vi "stimulate_and_record.vi"(3 "SSH password":string, 4 "Transfer and Run Date Folder After Experiment":bool, 5 "SSH user name":string, 6 "Tags":string, 7 "Frames":i32, 8 "Convert Power to Voltage":bool, 9 "voltages/power":dbl[](array[numeric]), 10 "parameters":string[](array[string]), 11 "parameters headers":string[](array[string])) -> ()   [LabVIEW 2014]
uses:
  <vilib>/userdefined/High Color/IMAQdx.ctl
  <vilib>/Utility/file.llb/Write To Spreadsheet File (DBL).vi
  <vilib>/Utility/file.llb/Write To Spreadsheet File (string).vi
  <vilib>/Utility/file.llb/Read From Spreadsheet File (string).vi
  <vilib>/vision/driver/NI_Vision_Acquisition_Software.lvlib
panel:
  out "JPEG Quality":dbl
  out "Error":string
  out "Save Directory":path
  out "Buffer Number Out":u32
  out "Image":T1(plugin-control)
  in  "stop":bool
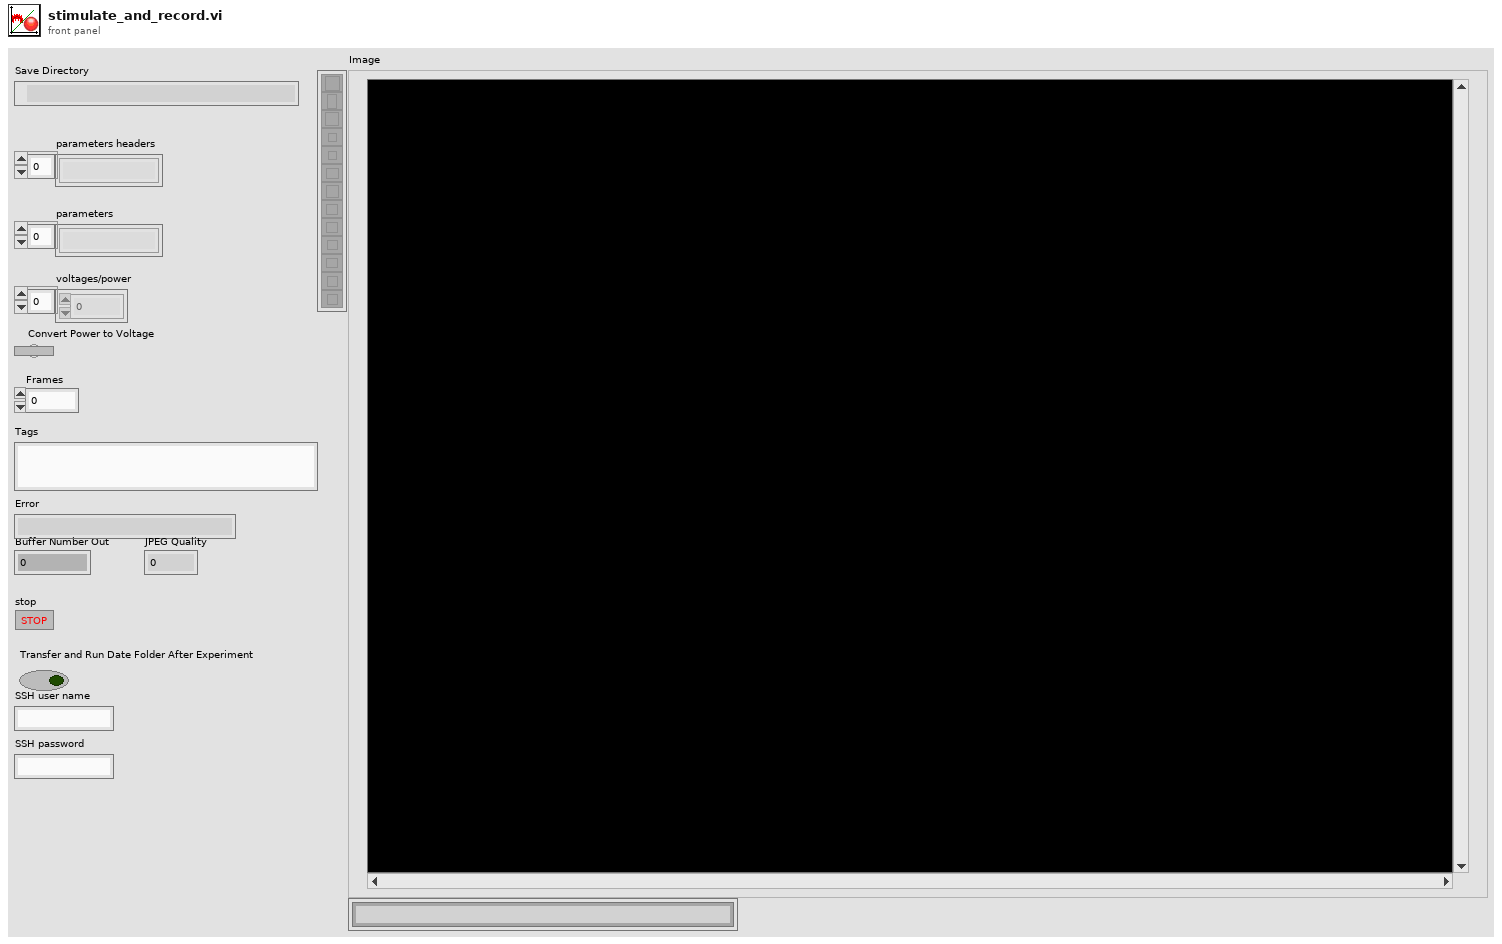
[diagram p1: front panel]
types:
  T1 = typedef "IMAQ Image.ctl" = refnum<image>
  T2 = typedef "IMAQdx.ctl" = refnum<k21>
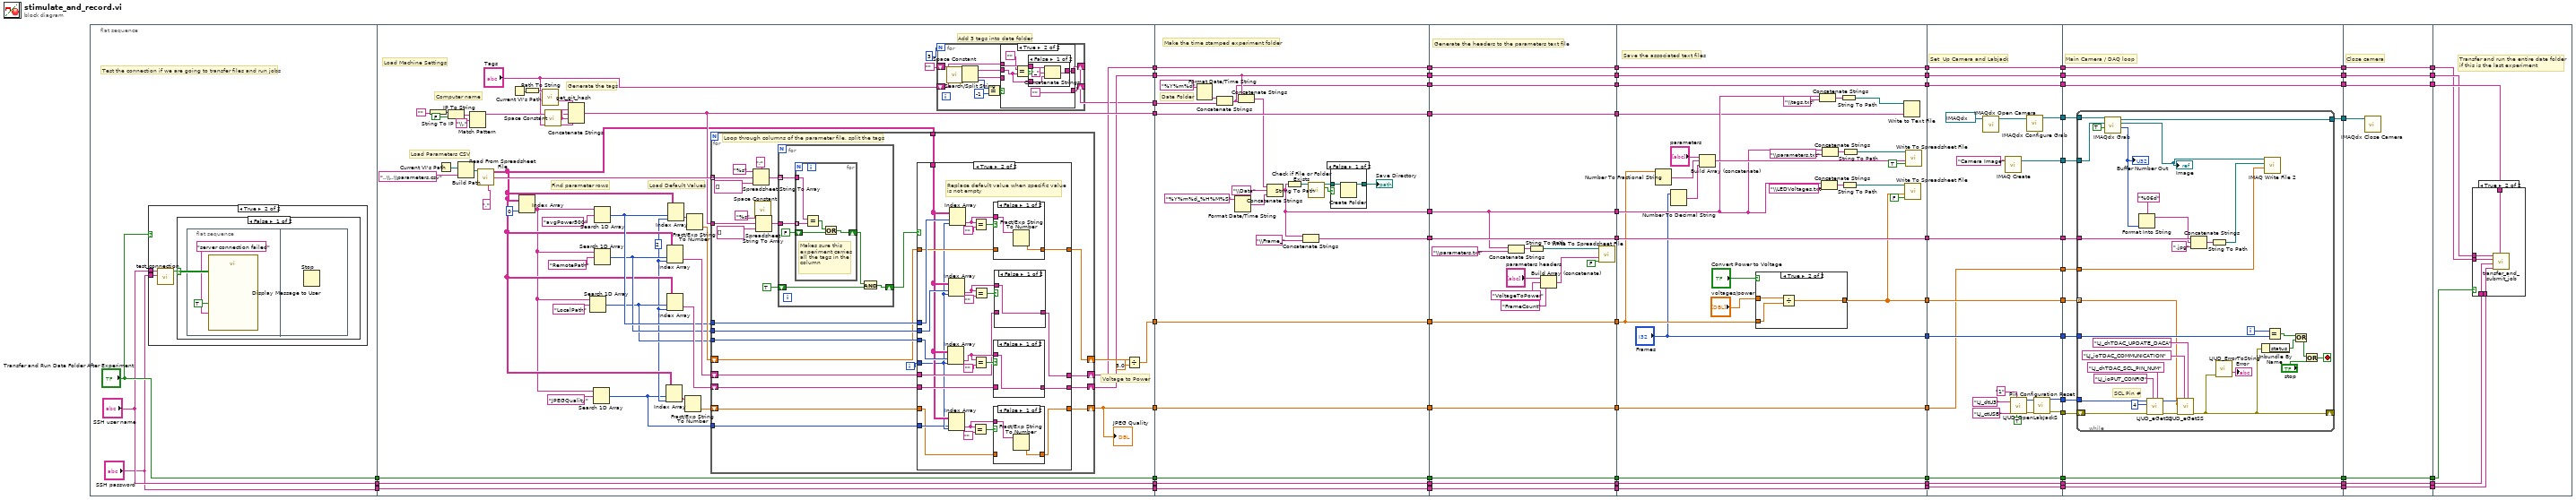
[diagram p0: block diagram]
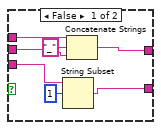
[diagram p4: hidden frame]
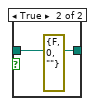
[diagram p11: hidden frame]
diagram:
  n1 = flat-sequence {
    tunnel: ["Transfer and Run Date Folder After Experiment"] -> w30
    tunnel: ["SSH user name"] -> w29
    tunnel: ["SSH password"] -> w28
    tunnel: [w118] -> w60
    tunnel: [w101] -> w59
    tunnel: [w92] -> w50
    tunnel: [w93] -> w49
    tunnel: w30 -> [w110]
    tunnel: w29 -> [w109]
    tunnel: w28 -> [w108]
    tunnel: [w110] -> w21
    tunnel: [w109] -> w14
    tunnel: [w108] -> w13
    tunnel: [w89] -> w6
    tunnel: [w80] -> w5
    tunnel: [w254] -> w44
    tunnel: [w253] -> w42
    tunnel: [w252] -> w40
    tunnel: [w251] -> w38
    tunnel: [w233] -> w36
    tunnel: [w235] -> w34
    tunnel: [w250] -> w32
    tunnel: w49 -> [w250]
    tunnel: w50 -> [w235]
    tunnel: w59 -> [w251]
    tunnel: w60 -> [w252]
    tunnel: [w242] -> w22
    tunnel: w21 -> [w242]
    tunnel: [w241] -> w15
    tunnel: w14 -> [w241]
    tunnel: w13 -> [w240]
    tunnel: [w240] -> w12
    tunnel: w6 -> [w236]
    tunnel: w5 -> [w232]
    tunnel: [w232] -> w1
    tunnel: w44 -> [w276]
    tunnel: [w276] -> w43
    tunnel: w42 -> [w262]
    tunnel: [w262] -> w41
    tunnel: w40 -> [w275]
    tunnel: [w275] -> w39
    tunnel: w38 -> [w274]
    tunnel: [w274] -> w37
    tunnel: w36 -> [w273]
    tunnel: [w273] -> w35
    tunnel: w34 -> [w272]
    tunnel: [w272] -> w33
    tunnel: w32 -> [w271]
    tunnel: [w271] -> w31
    tunnel: [w261] -> w23
    tunnel: w22 -> [w261]
    tunnel: [w260] -> w16
    tunnel: w15 -> [w260]
    tunnel: w12 -> [w259]
    tunnel: [w259] -> w11
    tunnel: [w258] -> w2
    tunnel: w1 -> [w258]
    tunnel: w43 -> [w304]
    tunnel: [w304] -> w65
    tunnel: [w287] -> w63
    tunnel: ["Frames"] -> w62
    tunnel: w41 -> [w296]
    tunnel: w39 -> [w283]
    tunnel: w37 -> [w278]
    tunnel: w35 -> [w292]
    tunnel: [w292] -> w55
    tunnel: [w291] -> w51
    tunnel: w33 -> [w291]
    tunnel: [w290] -> w45
    tunnel: w31 -> [w290]
    tunnel: [w281] -> w24
    tunnel: w23 -> [w281]
    tunnel: [w280] -> w17
    tunnel: w16 -> [w280]
    tunnel: w11 -> [w279]
    tunnel: [w279] -> w10
    tunnel: [w277] -> w3
    tunnel: w2 -> [w277]
    tunnel: w65 -> [w328]
    tunnel: [w330] -> w71
    tunnel: [w329] -> w70
    tunnel: [w328] -> w69
    tunnel: [w320] -> w67
    tunnel: [w319] -> w66
    tunnel: [w324] -> w64
    tunnel: w63 -> [w324]
    tunnel: w62 -> [w323]
    tunnel: [w323] -> w61
    tunnel: [w317] -> w56
    tunnel: w55 -> [w317]
    tunnel: [w316] -> w52
    tunnel: w51 -> [w316]
    tunnel: [w315] -> w46
    tunnel: w45 -> [w315]
    tunnel: [w314] -> w25
    tunnel: w24 -> [w314]
    tunnel: [w313] -> w18
    tunnel: w17 -> [w313]
    tunnel: w10 -> [w312]
    tunnel: [w312] -> w9
    tunnel: [w311] -> w4
    tunnel: w3 -> [w311]
    tunnel: w71 -> [w348]
    tunnel: w70 -> [w347]
    tunnel: w69 -> [w346]
    tunnel: [w345] -> w68
    tunnel: w67 -> [w344]
    tunnel: w66 -> [w343]
    tunnel: w64 -> [w342]
    tunnel: w61 -> [w341]
    tunnel: [w340] -> w57
    tunnel: w56 -> [w340]
    tunnel: [w339] -> w53
    tunnel: w52 -> [w339]
    tunnel: [w338] -> w47
    tunnel: w46 -> [w338]
    tunnel: [w337] -> w26
    tunnel: w25 -> [w337]
    tunnel: [w336] -> w19
    tunnel: w18 -> [w336]
    tunnel: w9 -> [w335]
    tunnel: [w335] -> w8
    tunnel: w4 -> [w334]
    tunnel: w68 -> [w387]
    tunnel: [w386] -> w58
    tunnel: w57 -> [w386]
    tunnel: [w385] -> w54
    tunnel: w53 -> [w385]
    tunnel: [w384] -> w48
    tunnel: w47 -> [w384]
    tunnel: [w383] -> w27
    tunnel: w26 -> [w383]
    tunnel: [w382] -> w20
    tunnel: w19 -> [w382]
    tunnel: w8 -> [w381]
    tunnel: [w381] -> w7
    tunnel: w58 -> [w393]
    tunnel: w54 -> [w392]
    tunnel: w48 -> [w391]
    tunnel: w27 -> [w390]
    tunnel: w20 -> [w389]
    tunnel: w7 -> [w388]
    frame #0 {
      # "Test the connection if we are going to transfer files and run jobs"
      n2 = case shown="True" "Transfer and Run Date Folder After Experiment" {
        tunnel: "SSH password" -> [_ w77]
        tunnel: "SSH user name" -> [_ w75]
        frame False {
        }
        frame True {
          n3 = call "test_connection.vi"("Username"=w75, "Password"=w77) -> ("Connection Successful"=w76:bool)  [unwired: 7 in]
          n4 = case shown="False" w76 {
            frame False {
              n5 = flat-sequence {
                frame #0 {
                  n6 = call "Display Message to User"("Enable"=TRUE, "Message"="server connection failed") -> ()  [unwired: 8 in, 2 out]
                }
                frame #1 {
                  n7 = Stop() -> ()  [unwired: 1 in]
                }
              }
            }
            frame True {
            }
          }
        }
      }
    }
    frame #1 {
      w83 = 2
      # "Add 3 tags into date folder"
      # "Generate the tags"
      # "Find parameter rows"
      # "Load Default Values"
      # "Voltage to Power"
      # "Load Parameters CSV"
      # "Computer name"
      # "Load Machine Settings"
      n8 = String To IP(1:"") -> (0:w126:u32)
      n9 = Current VI's Path() -> (path=w121:path)
      n10 = IP To String(1:FALSE, 2:w126) -> (0:w123:string)
      n11 = Build Path(base path=w121, name or relative path="..\\..\\parameters.csv") -> (appended path=w112:path)
      n12 = Match Pattern(string=w123, regular expression="\\.") -> (before substring=w103:string)  [unwired: 1 in, 3 out]
      n13 = call-poly <vilib>:"Read From Spreadsheet File.vi"("delimiter (\\t)"=",", "file path (dialog if empty)"=w112) -> ("first row"=w102:string[], "all rows"=w85:string[][])  [unwired: 5 in, 3 out]
      n14 = Current VI's Path() -> (path=w105:path)
      n15 = Index Array(array=w85, index (col)=0) -> (element=w84:string[])  [unwired: 1 in]
      n16 = Path To String(path=w105) -> (string=w104:string)
      n17 = call "get_git_hash.vi"("VI folder"=w104) -> ("github hash"=w107:string)  [unwired: 10 in]
      n18 = call <vilib>:"Space Constant.vi"() -> ("String"=w106:string)
      n19 = Concatenate Strings(w107, w106, w103, w106, "Tags") -> (w101:string)
      n20 = Search 1D Array(1D array=w84, element="LocalPath") -> (index of element=w95:i32)  [unwired: 1 in]
      n21 = Search 1D Array(1D array=w84, element="JPEGQuality") -> (index of element=w81:i32)  [unwired: 1 in]
      n22 = Search 1D Array(1D array=w84, element="RemotePath") -> (index of element=w96:i32)  [unwired: 1 in]
      n23 = Search 1D Array(1D array=w84, element="avgPower500") -> (index of element=w97:i32)  [unwired: 1 in]
      n24 = Index Array(array=w85, index (row)=w81, index (col)=w83) -> (element=w86:string)
      n25 = Index Array(array=w85, index (row)=w96, index (col)=w83) -> (element=w99:string)
      n26 = Index Array(array=w85, index (row)=w95, index (col)=w83) -> (element=w98:string)
      n27 = Index Array(array=w85, index (row)=w97, index (col)=w83) -> (element=w114:string)
      n28 = Fract/Exp String To Number(string=w86) -> (number=w82:dbl)  [unwired: 3 in, 1 out]
      n29 = Fract/Exp String To Number(string=w114) -> (number=w100:dbl)  [unwired: 3 in, 1 out]
      n30 = for {
        tunnel: w102 -> [w180] mode=indexing
        tunnel: w101 -> [w172]
        tunnel: w97 -> [w167]
        tunnel: w96 -> [w166]
        tunnel: w95 -> [w165]
        tunnel: w85 -> [w170]
        shift-right: [w162] -> w94
        shift-left: w100 -> [w163]
        shift-right: [w159] -> w93
        shift-left: w99 -> [w160]
        shift-right: [w158] -> w92
        shift-left: w98 -> [w161]
        shift-right: [w155] -> w80
        shift-left: w82 -> [w157]
        tunnel: w81 -> [w156]
        i -> [w164]
        # "Loop through columns of the parameter file, split the tags"
        n31 = Spreadsheet String To Array(delimiter (Tab)=";", format string="%s", spreadsheet string=w180, array type (2D Dbl)=string[] []) -> (array=w176:string[])
        n32 = call <vilib>:"Space Constant.vi"() -> ("String"=w174:string)
        n33 = Spreadsheet String To Array(delimiter (Tab)=w174, format string="%s", spreadsheet string=w172, array type (2D Dbl)=string[] []) -> (array=w171:string[])
        n34 = for {
          tunnel: w176 -> [w226] mode=indexing
          tunnel: w171 -> [w225]
          shift-right: [w223] -> w168
          shift-left: TRUE -> [w221]
          n35 = for {
            tunnel: w226 -> [w231]
            tunnel: w225 -> [w230] mode=indexing
            shift-right: [w227] -> w222
            shift-left: FALSE -> [w228]
            # "Makes sure this\nexperiment carries\nall the tags in the\ncolumn"
            n36 = Equal?(x=w231, y=w230) -> (x = y?=w229:bool)
            n37 = Or(x=w229, y=w228) -> (x .or. y?=w227:bool)
          }
          n38 = And(x=w222, y=w221) -> (x .and. y?=w223:bool)
        }
        n39 = case shown="True" w168 {
          tunnel: w163 -> [w184 w205]
          tunnel: [w184 w204] -> w162
          tunnel: w167 -> [_ w210]
          tunnel: w166 -> [_ w209]
          tunnel: w165 -> [_ w208]
          tunnel: w164 -> [_ w187]
          tunnel: w170 -> [_ w188]
          tunnel: [w183 w194] -> w159
          tunnel: [w182 w196] -> w158
          tunnel: w161 -> [w182 w195]
          tunnel: w160 -> [w183 w193]
          tunnel: w157 -> [w181 w185]
          tunnel: w156 -> [_ w186]
          tunnel: [w181 w189] -> w155
          frame False {
          }
          frame True {
            # "Replace default value when specific value\nis not empty"
            n40 = Index Array(array=w188, index (row)=w208, index (col)=w187) -> (element=w197:string)
            n41 = Index Array(array=w188, index (row)=w209, index (col)=w187) -> (element=w200:string)
            n42 = Index Array(array=w188, index (row)=w186, index (col)=w187) -> (element=w190:string)
            n43 = Index Array(array=w188, index (row)=w210, index (col)=w187) -> (element=w203:string)
            n44 = Equal?(x=w190, y="") -> (x = y?=w191:bool)
            n45 = Equal?(x=w203, y="") -> (x = y?=w206:bool)
            n46 = Equal?(x=w197, y="") -> (x = y?=w198:bool)
            n47 = Equal?(x=w200, y="") -> (x = y?=w201:bool)
            n48 = case shown="False" w191 {
              tunnel: w185 -> [_ w213]
              tunnel: [w212 w213] -> w189
              tunnel: w190 -> [w211 _]
              frame False {
                n49 = Fract/Exp String To Number(string=w211) -> (number=w212:dbl)  [unwired: 3 in, 1 out]
              }
              frame True {
              }
            }
            n50 = case shown="False" w206 {
              tunnel: w205 -> [_ w220]
              tunnel: [w219 w220] -> w204
              tunnel: w203 -> [w218 _]
              frame False {
                n51 = Fract/Exp String To Number(string=w218) -> (number=w219:dbl)  [unwired: 3 in, 1 out]
              }
              frame True {
              }
            }
            n52 = case shown="False" w198 {
              tunnel: w197 -> [w214 _]
              tunnel: [w214 w215] -> w196
              tunnel: w195 -> [_ w215]
              frame False {
              }
              frame True {
              }
            }
            n53 = case shown="False" w201 {
              tunnel: w200 -> [w216 _]
              tunnel: [w216 w217] -> w194
              tunnel: w193 -> [_ w217]
              frame False {
              }
              frame True {
              }
            }
          }
        }
      }
      "JPEG Quality" <- w80
      n54 = for {
        N: 3 -> [_]
        shift-right: [w127] -> _
        shift-left: "Tags" -> [w136]
        shift-right: [w129] -> w89
        shift-left: "" -> [w134]
        n55 = call <vilib>:"Space Constant.vi"() -> ("String"=w135:string)
        n56 = Search/Split String(string=w136, search string/char (-)=w135) -> (substring before match=w133:string, match + rest of string=w132:string, offset of match=w131:i32)  [unwired: 1 in]
        n57 = Equal?(x=w131, y=-1) -> (x = y?=w128:bool)
        n58 = case shown="True" w128 {
          tunnel: w134 -> [w137 w147]
          tunnel: w133 -> [w138 w144]
          tunnel: w132 -> [w139 _]
          tunnel: [w141 ""] -> w127
          tunnel: [w140 w146] -> w129
          frame False {
            n59 = String Subset(string=w139, offset (0)=1) -> (substring=w141:string)  [unwired: 1 in]
            n60 = Concatenate Strings(w137, "_", w138) -> (w140:string)
          }
          frame True {
            n61 = Equal?(x="", y=w144) -> (x = y?=w148:bool)
            n62 = case shown="False" w148 {
              tunnel: w147 -> [w151 w154]
              tunnel: [w152 w154] -> w146
              tunnel: w144 -> [w150 _]
              frame False {
                n63 = Concatenate Strings(w151, "_", w150) -> (w152:string)
              }
              frame True {
              }
            }
          }
        }
      }
      n64 = Divide(x=w94, y=5.0) -> (x/y=w118:dbl)
    }
    frame #2 {
      # "Make the time stamped experiment folder"
      # "Date Folder"
      n65 = Format Date/Time String(time format string (%c)="%Y%m%d") -> (date/time string=w237:string)  [unwired: 2 in]
      n66 = Concatenate Strings(w237, w236) -> (w233:string)
      n67 = Format Date/Time String(time format string (%c)="%Y%m%d_%H%M%S") -> (date/time string=w239:string)  [unwired: 2 in]
      n68 = Concatenate Strings(w235, w233) -> (w234:string)
      n69 = Concatenate Strings(w234, "\\Data", w239) -> (w253:string)
      n70 = String To Path(string=w253) -> (path=w245:path)
      n71 = Concatenate Strings(w253, "\\Frame_") -> (w254:string)
      n72 = call <vilib>:"Check if File or Folder Exists.vi"("path"=w245) -> ("file or folder exists?"=w248:bool, "dup path"=w247:path)  [unwired: 8 in, 1 out]
      n73 = case shown="False" w248 {
        tunnel: [w255 w257] -> w244
        tunnel: w247 -> [w256 w257]
        frame False {
          n74 = Create Folder(path (use dialog)=w256) -> (created path=w255:path)  [unwired: 2 in, 2 out]
        }
        frame True {
          (unwired) errorcluster {"status"=FALSE, "code"=0, "source"=""} ("error out")
        }
      }
      "Save Directory" <- w244
    }
    frame #3 {
      # "Generate the headers to the parameters text file"
      n75 = Concatenate Strings(w262, "\\parameters.txt") -> (w270:string)
      n76 = String To Path(string=w270) -> (path=w269:path)
      n77 = Build Array (concatenate)("parameters headers", "VoltageToPower", "FrameCount") -> (w266:string[])
      n78 = call-poly <vilib>:"Write To Spreadsheet File.vi"("append to file? (new file:F)"=FALSE, "1D data"=w266, "file path (dialog if empty)"=w269) -> ()  [unwired: 5 in, 1 out]
    }
    frame #4 {
      # "Save the associated text files"
      n79 = Number To Fractional String(number=w283) -> (F-format string=w284:string)  [unwired: 3 in]
      n80 = Number To Decimal String(number="Frames") -> (decimal integer string=w285:string)  [unwired: 1 in]
      n81 = Build Array (concatenate)("parameters", w284, w285) -> (w297:string[])
      n82 = case shown="True" "Convert Power to Voltage" {
        tunnel: "voltages/power" -> [w307 w310]
        tunnel: [w307 w308] -> w287
        tunnel: w283 -> [_ w309]
        frame False {
        }
        frame True {
          n83 = Divide(x=w310, y=w309) -> (x/y=w308:dbl[])
        }
      }
      n84 = Concatenate Strings(w296, "\\tags.txt") -> (w294:string)
      n85 = Concatenate Strings(w296, "\\LEDVoltages.txt") -> (w306:string)
      n86 = Concatenate Strings(w296, "\\parameters.txt") -> (w301:string)
      n87 = String To Path(string=w294) -> (path=w293:path)
      n88 = String To Path(string=w306) -> (path=w305:path)
      n89 = String To Path(string=w301) -> (path=w300:path)
      n90 = Write to Text File(file (use dialog)=w293, text=w278) -> ()  [unwired: 2 in, 3 out]
      n91 = call-poly <vilib>:"Write To Spreadsheet File.vi"("append to file? (new file:F)"=FALSE, "1D data"=w287, "file path (dialog if empty)"=w305) -> ()  [unwired: 5 in, 1 out]
      n92 = call-poly <vilib>:"Write To Spreadsheet File.vi"("append to file? (new file:F)"=TRUE, "1D data"=w297, "file path (dialog if empty)"=w300) -> ()  [unwired: 5 in, 1 out]
    }
    frame #5 {
      # "Set  Up Camera and Labjack"
      n93 = call <vilib>:"IMAQdx Open Camera.vi"("Session In"=T2 "cam0") -> ("Session Out"=w332:T2)  [unwired: 9 in, 1 out]
      n94 = call "IMAQ Create"("Image Name"="Camera Image") -> ("New Image"=w329:T1)  [unwired: 4 in, 1 out]
      n95 = call "LJUD_OpenLabJackS.vi"("FirstFound"=TRUE, "Address"="1" ("DeviceType"), "ConnectionType"="LJ_ctUSB", "DeviceType"="LJ_dtU3") -> ("error out"=w318:errorcluster, "Handle"=w321:i32)  [unwired: 5 in, 1 out]
      n96 = call <vilib>:"IMAQdx Configure Grab.vi"("Session In"=w332) -> ("Session Out"=w330:T2)  [unwired: 9 in, 1 out]
      n97 = call "Pin Configuration Reset.vi"("error in"=w318, "Handle In"=w321) -> ("error out"=w319:errorcluster, "Handle Out"=w320:i32)  [unwired: 8 in]
    }
    frame #6 {
      # "Main Camera / DAQ loop"
      n98 = while {
        tunnel: w348 -> [w380]
        tunnel: [w379] -> w345
        tunnel: w347 -> [w378]
        tunnel: w346 -> [w376]
        tunnel: w344 -> [w353]
        shift-right: [w354] -> _
        shift-left: w343 -> [w352]
        tunnel: w342 -> [w351] mode=indexing
        tunnel: w341 -> [w362]
        tunnel: w334 -> [w350]
        i -> [w363]
        stop <- w369 stop-if-true
        # "SCL Pin #"
        n99 = call <vilib>:"IMAQdx Grab.vi"("Wait for Next Buffer? (Yes)"=TRUE, "Image In"=w378, "Session In"=w380) -> ("Buffer Number Out"=w372:u32, "Image Out"=w377:T1, "Session Out"=w379:T2)  [unwired: 5 in, 1 out]
        "Image" <- w377
        "Buffer Number Out" <- w372
        n100 = Format Into String(format string="%06d" ("string"), w372) -> (resulting string=w371:string)  [unwired: 2 in, 1 out]
        n101 = call "LJUD_eGetSS.vi"("Channel"="LJ_chTDAC_SCL_PIN_NUM", "IOType"="LJ_ioPUT_CONFIG", "error in"=w352, "Value Write"=4, "Handle In"=w353) -> ("error out"=w355:errorcluster, "Handle Out"=w358:i32)  [unwired: 4 in, 1 out]
        n102 = call "LJUD_eGetSS.vi"("Channel"="LJ_chTDAC_UPDATE_DACA", "IOType"="LJ_ioTDAC_COMMUNICATION", "error in"=w355, "Value Write"=w351, "Handle In"=w358) -> ("error out"=w354:errorcluster)  [unwired: 4 in, 2 out]
        n103 = Concatenate Strings(w376, w371, ".jpg" ("string")) -> (w374:string)
        n104 = String To Path(string=w374) -> (path=w373:path)
        n105 = call "LJUD_ErrorToString.vi"("error in"=w354) -> ("String"=→"Error":string)  [unwired: 10 in]
        n106 = Unbundle By Name(w354) -> ("status"=w366:bool)
        n107 = call-poly "IMAQ Write File 2"("Image Quality"=w350, "File Path"=w373, "Image"=w377) -> ()  [unwired: 7 in, 2 out]
        n108 = Equal?(x=w363, y=w362) -> (x = y?=w365:bool)
        n109 = Or(x=w365, y=w366) -> (x .or. y?=w364:bool)
        n110 = Or(x=w364, y="stop") -> (x .or. y?=w369:bool)
      }
    }
    frame #7 {
      # "Close camera"
      n111 = call <vilib>:"IMAQdx Close Camera.vi"("Session In"=w387) -> ()  [unwired: 10 in, 1 out]
    }
    frame #8 {
      # "Transfer and run the entire date folder\nif this is the last experiment"
      n112 = case shown="True" w390 {
        tunnel: w393 -> [_ w398]
        tunnel: w392 -> [_ w397]
        tunnel: w391 -> [_ w396]
        tunnel: w389 -> [_ w395]
        tunnel: w388 -> [_ w394]
        frame False {
        }
        frame True {
          n113 = call "transfer_and_submit_job.vi"("Date Folder"=w398, "Password"=w394, "Username"=w395, "Remote Data Directory"=w396, "Local Data Directory"=w397) -> ()  [unwired: 7 in]
        }
      }
    }
  }
